vi "captureSpectImage.vi"(8 "error in (no error)":errorcluster, 10 "command_captureSpectImage":T1, 11 "Model in":refnum<class "Model.lvclass">) -> (0 "error out":errorcluster, 3 "Model out":refnum<class "Model.lvclass">)   [LabVIEW 2016, in "Model.lvclass"]
uses:
  Model.lvclass
  ts_sallv_FiberSpectrograph/DataTypes/command_captureSpectImage.ctl
  Model.lvclass/Model.ctl
  ss_sedspectrometer/SEDSpectrometer/FiberSpectrograph.lvclass
  ts_sallv_FiberSpectrograph/SALLV_FiberSpectrograph.lvlib
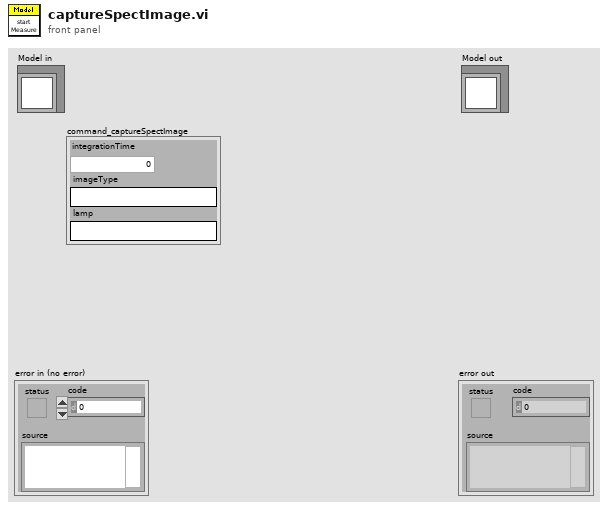
[diagram p1: front panel]
types:
  T1 = typedef "SALLV_FiberSpectrograph.lvlib/command_captureSpectImage.ctl" = cluster{"integrationTime":sgl, "imageType":string, "lamp":string}
  T2 = cluster{"StartPixel":u16, "StopPixel":u16, "IntegrationTime":sgl, "IntegrationDelay":u32, "NrAverages":u32, "DarkCorrectionType":cluster{"Enable CorDynDark":u8, "ForgetPercentage":u8}, "SmoothingType":cluster{"SmoothPix":u16, "SmoothModel":u8}, "SatDetection":u8, "TriggerType":cluster{"Trigger Mode":u8, "Trigger Source":u8, "Trigger SourceType":u8}, "ControlSettingsType":cluster{"StrobeControl":u16, "LaserDelay":u32, "LaserWidth":u32, "LaserWaveLength":sgl, "StoreToRam":u16}}
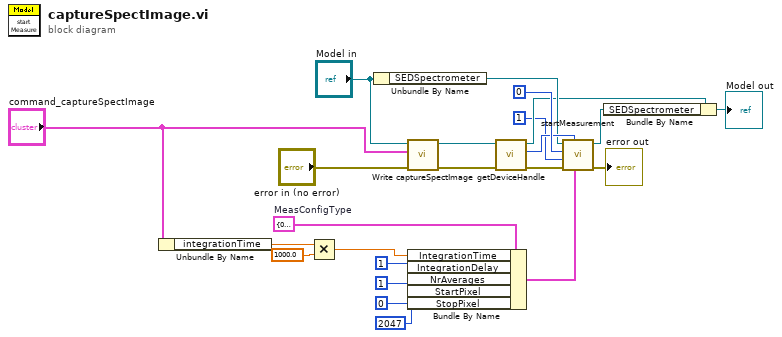
[diagram p0: block diagram]
diagram:
  w23 = T2 {"StartPixel"=0, "StopPixel"=0, "IntegrationTime"=0.0, "IntegrationDelay"=0, "NrAverages"=0, "DarkCorrectionType"={"Enable CorDynDark"=0, "ForgetPercentage"=0}, "SmoothingType"={"SmoothPix"=0, "SmoothModel"=0}, "SatDetection"=0, "TriggerType"={"Trigger Mode"=0, "Trigger Source"=0, "Trigger SourceType"=0}, "ControlSettingsType"={"StrobeControl"=0, "LaserDelay"=0, "LaserWidth"=0, "LaserWaveLength"=0.0, "StoreToRam"=0}}  # MeasConfigType
  n1 = Unbundle By Name("command_captureSpectImage") -> ("integrationTime"=w9:sgl)
  n2 = Multiply(x=w9, y=sgl 1000.0) -> (x*y=w7:sgl)
  n3 = Unbundle By Name("Model in") -> ("SEDSpectrometer"=w16:refnum<class "FiberSpectrograph.lvclass">)
  n4 = call-dynamic "Write captureSpectImage.vi"("error in (no error)"="error in (no error)", "command_captureSpectImage"="command_captureSpectImage", "Model in"="Model in") -> ("error out"=w2:errorcluster, "Model out"=w1:refnum<class "Model.lvclass">)  [unwired: 7 in]
  n5 = Bundle By Name(cluster=w23, "IntegrationTime"=w7, "IntegrationDelay"=u32 1, "NrAverages"=u32 1, "StartPixel"=u16 0, "StopPixel"=u16 2047) -> (w20:T2)
  n6 = call-dynamic "getDeviceHandle.vi"("error in (no error)"=w2, "Model in"=w1) -> ("error out"=w17:errorcluster, "Device"=w18:i32, "Model out"=w15:refnum<class "Model.lvclass">)  [unwired: 7 in]
  n7 = call "startMeasurement.vi"("MeasConfigType"=w20, "Device Handle"=w18, "error in (no error)"=w17, "NumOfScans"=i16 1, "a_hWnd"=0, "SEDSpectrometer in"=w16) -> ("error out"=→"error out":errorcluster, "SEDSpectrometer out"=w13:refnum<class "FiberSpectrograph.lvclass">)  [unwired: 2 in, 2 out]
  n8 = Bundle By Name(cluster=w15, "SEDSpectrometer"=w13) -> (→"Model out":refnum<class "Model.lvclass">)
